vi "SF_app_IC_de_X_1D_enonce.vi"() -> ()   [LabVIEW 2010]
panel:
  in  "Niveau de confiance avec":u16(ring) items=["Risque alpha bilattéral", "Risque alpha à droite", "Risque alpha à gauche"]
  in  "Niveau de confiance\n= 1- alpha":dbl
  out "taille n échantillon":i32
  out "sigma pop estimé":dbl caption="écart-type estimé population\nSigma_pop" format="%0.2f"
  out "x_bar":dbl caption="moyenne\nechantillon\n(x_bar)" format="%0.2f"
  in  "Données de l'échantillon":dbl[](array[numeric])
  out "Ic max":dbl
  out "Ic min":dbl
  out "sigma x_bar":dbl
  # "Palette Maths.Probabilités et statistiques\nVariance et écart-type\nCâbler la commande Pondération.\nSélectionner Sample quand X est un échantillon, et Population quand X contient toutes les valeurs de la population\nAvec Sample, l'écart-type calculé est pondéré par Racine(n/n-1), n étant le nombre de valeurs de l'échantillon"
  # "Palette Maths.Probabilités et Statistiques.Probabilités\nCDF inverse continue.\nSélectionner loi normale\nMoyenne de 0\nEcart-type de 1\nOn obtient la valeur de t pour avoir F(t)=alpha/2"
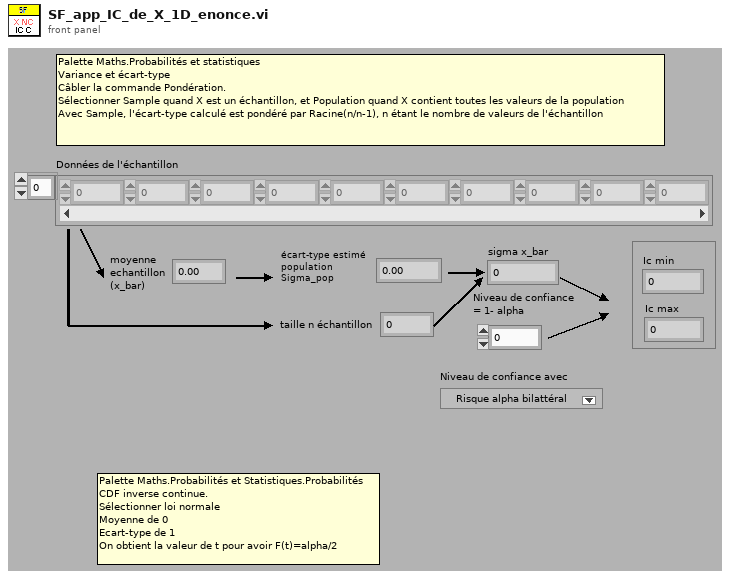
[diagram p1: front panel]
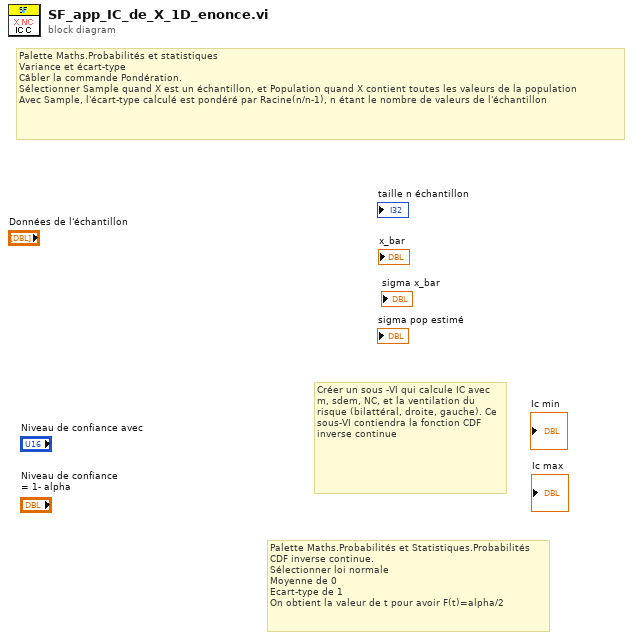
[diagram p0: block diagram]
diagram:
  # "Créer un sous -VI qui calcule IC avec \nm, sdem, NC, et la ventilation du risque (bilattéral, droite, gauche). Ce sous-VI contiendra la fonction CDF inverse continue"
  # "Palette Maths.Probabilités et statistiques\nVariance et écart-type\nCâbler la commande Pondération.\nSélectionner Sample quand X est un échantillon, et Population quand X contient toutes les valeurs de la population\nAvec Sample, l'écart-type calculé est pondéré par Racine(n/n-1), n étant le nombre de valeurs de l'échantillon"
  # "Palette Maths.Probabilités et Statistiques.Probabilités\nCDF inverse continue.\nSélectionner loi normale\nMoyenne de 0\nEcart-type de 1\nOn obtient la valeur de t pour avoir F(t)=alpha/2"
